vi "Strip Path X Times.vi"(9 "# to Strip(2)":i32=2, 11 "Path":path) -> (1 "Stripped Path names":string[](array[string]), 3 "Stripped Path":path)   [LabVIEW 2011]
doc: "This VI will strip the input path the number of times indicated in # to Strip input. The Stripped Path names output will contain an array of the paths that were stripped."
panel:
  # "Strip Path X Times.vi\n\nThis adds the useful option of sepecifing the number of times to strip a path\nto the \"Strip Path\" primitive.\n\nCopyright (C) 2003 Edwin Dickens  edwind@distek.com\n\nPlease visit http://www.OpenG.org to learn about the\nOpen Source LabVIEW software movement.\n\nThis library is free software; you can redistribute it and/or\nmodify it under the terms of the GNU Lesser General Public\nLicense as published by the Free Software Foundation; either\nversion 2.1 of the License, or (at your option) any later version.\nThis library is distributed in the hope that it will be useful,\nbut WITHOUT ANY WARRANTY; without even the implied warranty of\nMERCHANTABILITY or FITNESS FOR A PARTICULAR PURPOSE. See the GNU\nLesser General Public License for more details.\nYou should have received a copy of the GNU Lesser General Public\nLicense along with this library; if not, write to the Free Software\nFoundation, Inc., 59 Temple Place, Suite 330, Boston, MA 02111-1307 USA"
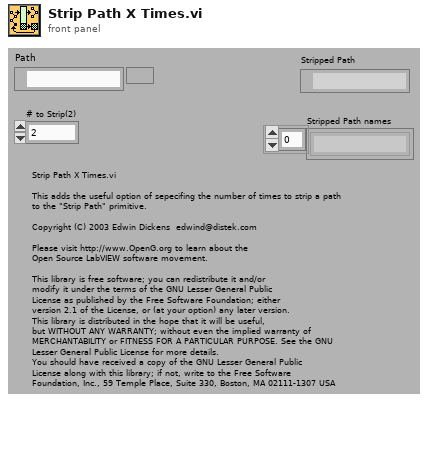
[diagram p1: front panel]
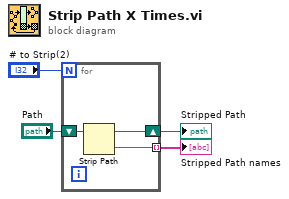
[diagram p0: block diagram]
diagram:
  n1 = for {
    N: "# to Strip(2)" -> [_]
    shift-right: [w6] -> w3
    shift-left: "Path" -> [w7]
    tunnel: [w5] -> w1 mode=indexing
    n2 = Strip Path(path=w7) -> (stripped path=w6:path, name=w5:string)
  }
  "Stripped Path" <- w3
  "Stripped Path names" <- w1
